vi "SCT Has Variable Changed.vi"(1 "changes":T1, 2 "Variable":T4) -> (0 "Boolean":bool)   [LabVIEW 2016]
uses:
  <resource>/dialog/variable/SCT Variable.ctl
  <vilib>/variable/Type Descriptor.ctl
  <vilib>/variable/Attribs.ctl
  <resource>/dialog/variable/SCT Variable Changes.ctl
  <resource>/dialog/variable/SCT Attribute Changes.ctl
  <vilib>/variable/NI_Variable.lvlib
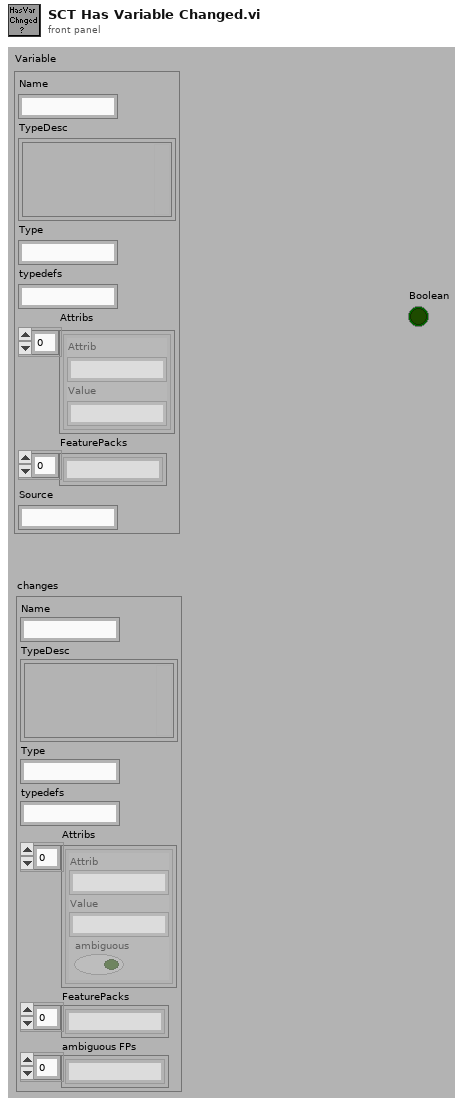
[diagram p1: front panel]
types:
  T1 = typedef "SCT Variable Changes.ctl" = cluster{"Name":string, "TypeDesc":T2, "Type":string, "typedefs":string, "Attribs":T3, "FeaturePacks":string[], "ambiguous FPs":string[]}
  T2 = typedef "NI_Variable.lvlib/Type Descriptor.ctl" = cluster{"Variant":variant}
  T3 = typedef "SCT Attribute Changes.ctl" = cluster{"Attrib":string, "Value":string, "ambiguous":bool}[]
  T4 = typedef "SCT Variable.ctl" = cluster{"Name":string, "TypeDesc":T2, "Type":string, "typedefs":string, "Attribs":T5, "FeaturePacks":string[], "Source":string}
  T5 = typedef "NI_Variable.lvlib/Attribs.ctl" = cluster{"Attrib":string, "Value":string}[]
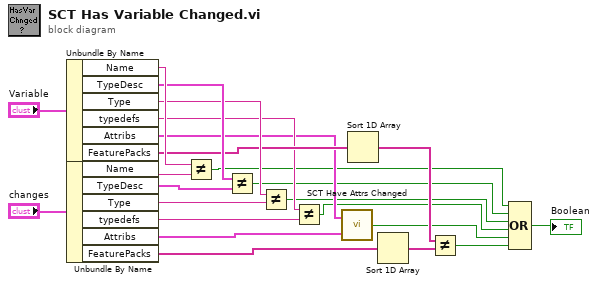
[diagram p0: block diagram]
diagram:
  n1 = Unbundle By Name("Variable") -> ("Name"=w22:string, "TypeDesc"=w21:T2, "Type"=w20:string, "typedefs"=w14:string, "Attribs"=w10:T5, "FeaturePacks"=w19:string[])
  n2 = Unbundle By Name("changes") -> ("Name"=w17:string, "TypeDesc"=w16:T2, "Type"=w15:string, "typedefs"=w13:string, "Attribs"=w11:T3, "FeaturePacks"=w12:string[])
  n3 = Not Equal?(x=w22, y=w17) -> (x != y?=w2:bool)
  n4 = Not Equal?(x=w21, y=w16) -> (x != y?=w3:bool)
  n5 = Not Equal?(x=w20, y=w15) -> (x != y?=w4:bool)
  n6 = Not Equal?(x=w14, y=w13) -> (x != y?=w5:bool)
  n7 = call <resource>:"SCT Have Attrs Changed.vi"("Attrib Changes"=w11, "Attribs"=w10) -> ("Boolean"=w6:bool)
  n8 = Sort 1D Array(array=w19) -> (sorted array=w8:string[])
  n9 = Sort 1D Array(array=w12) -> (sorted array=w7:string[])
  n10 = Not Equal?(x=w8, y=w7) -> (x != y?=w9:bool)
  n11 = Compound Arithmetic op=OR(w2, w3, w4, w5, w6, w9) -> (→"Boolean":bool)
